vi "Get Child Classes.vi"(8 "error in (no error)":errorcluster, 11 "Test in":refnum<class "Test.lvclass">) -> (0 "error out":errorcluster, 2 "Child Classes":refnum<class "Test.lvclass">[](array[class]))   [LabVIEW 2018, in "Test.lvclass"]
uses:
  Test.lvclass
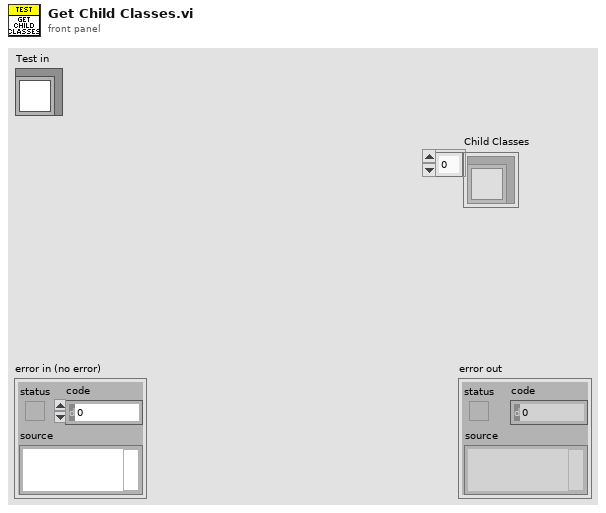
[diagram p1: front panel]
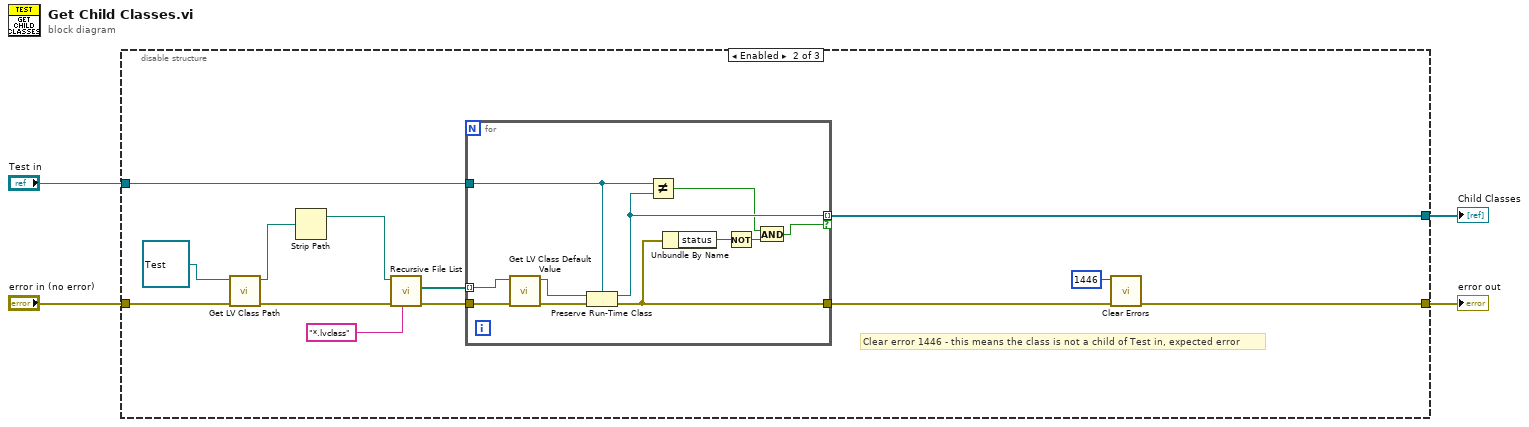
[diagram p0: block diagram]
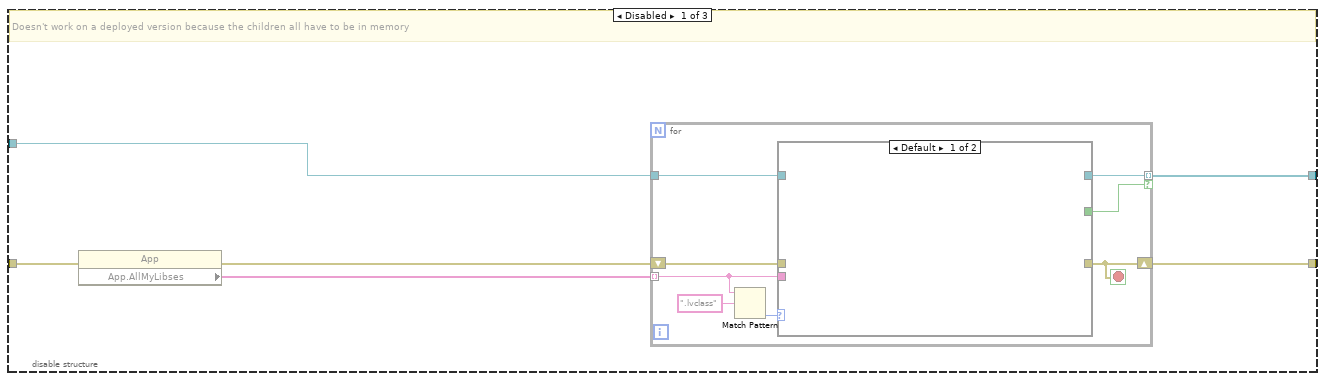
[diagram p2: hidden frame]
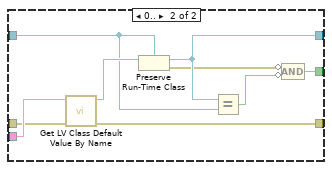
[diagram p3: hidden frame]
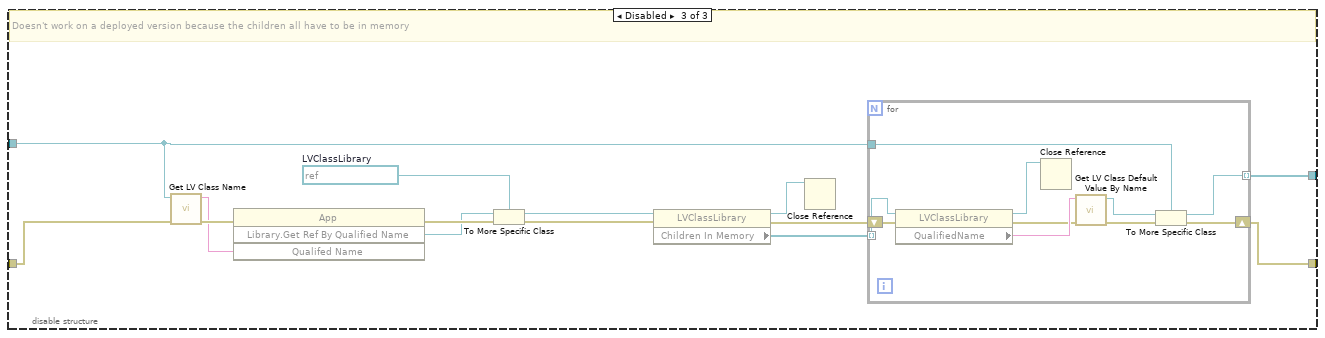
[diagram p4: hidden frame]
diagram:
  n1 = disable-structure shown="Enabled" {
    disable-tunnel: "Test in" -> [w8 w32 w52]
    disable-tunnel: [w7 w31 w53] -> w3
    disable-tunnel: "error in (no error)" -> [w6 w40 w55]
    disable-tunnel: [w5 w29 w54] -> w1
    frame Disabled {
      # "Doesn't work on a deployed version because the children all have to be in memory"
      n2 = property class="App"(error in=w6) -> (error out=w9:errorcluster, "App.AllMyLibses"=w10:string[])  [unwired: 1 in, 1 out]
      n3 = for {
        tunnel: w10 -> [w18] mode=indexing
        tunnel: [w13] -> w7 mode=indexing if=w12
        shift-right: [w14] -> w5
        shift-left: w9 -> [w15]
        tunnel: w8 -> [w11]
        stop <- w14 stop-if-true
        n4 = Match Pattern(string=w18, regular expression=".lvclass") -> (offset past match=w17:i32)  [unwired: 1 in, 3 out]
        n5 = case shown="Default" w17 {
          tunnel: [_ w26] -> w13
          tunnel: w18 -> [_ w23]
          tunnel: [_ w22] -> w12
          tunnel: [_ w21] -> w14
          tunnel: w15 -> [_ w20]
          tunnel: w11 -> [_ w19]
          frame Default {
          }
          frame 0.. {
            n6 = call <vilib>:"Get LV Class Default Value By Name.vi"("error in (no error)"=w20, "class name"=w23) -> ("error out"=w21:errorcluster, "object"=w27:refnum<class>)  [unwired: 8 in]
            n7 = Preserve Run-Time Class(object in=w27, 2:w19) -> (object out=w26:refnum<class "Test.lvclass">, error out=w24:errorcluster)  [unwired: 1 in]
            n8 = Equal?(x=w26, y=w19) -> (x = y?=w25:bool)
            n9 = Compound Arithmetic op=AND(invert w24, invert w25) -> (w22:bool)
          }
        }
      }
    }
    frame Enabled {
      # "Clear error 1446 - this means the class is not a child of Test in, expected error"
      n10 = call <vilib>:"Get LV Class Path.vi"("error in (no error)"=w40, "object"=refnum<class "Test.lvclass"> refnum ("Test.lvclass")) -> ("error out"=w36:errorcluster, "class path"=w39:path)  [unwired: 8 in]
      n11 = Strip Path(path=w39) -> (stripped path=w37:path)  [unwired: 1 out]
      n12 = call <vilib>:"Recursive File List.vi"("pattern"="*.lvclass", "error in (no error)"=w36, "Folder Path"=w37) -> ("error out"=w33:errorcluster, "All Files in Dir"=w34:path[])  [unwired: 4 in, 3 out]
      n13 = for {
        tunnel: w34 -> [w50] mode=indexing
        tunnel: w33 -> [w51]
        tunnel: w32 -> [w44]
        tunnel: [w45] -> w31 mode=indexing if=w41
        tunnel: [w47] -> w30
        n14 = call <vilib>:"Get LV Class Default Value.vi"("error in (no error)"=w51, "class path"=w50) -> ("error out"=w49:errorcluster, "object"=w48:refnum<class>)  [unwired: 8 in]
        n15 = Preserve Run-Time Class(object in=w48, error in=w49, 2:w44) -> (object out=w45:refnum<class "Test.lvclass">, error out=w47:errorcluster)
        n16 = Not Equal?(x=w44, y=w45) -> (x != y?=w42:bool)
        n17 = Unbundle By Name(w47) -> ("status"=w46:bool)
        n18 = Not(x=w46) -> (.not. x?=w43:bool)
        n19 = And(x=w42, y=w43) -> (x .and. y?=w41:bool)
      }
      n20 = call <vilib>:"Clear Errors.vi"("error in (no error)"=w30, "specific error code to clear (0: all)"=1446) -> ("error out"=w29:errorcluster)  [unwired: 4 in, 1 out]
    }
    frame Disabled {
      w56 = refnum<vi> refnum  # LVClassLibrary
      # "Doesn't work on a deployed version because the children all have to be in memory"
      n21 = call <vilib>:"Get LV Class Name.vi"("error in (no error)"=w55, "object"=w52) -> ("error out"=w58:errorcluster, "class name"=w57:string)  [unwired: 8 in]
      n22 = invoke class="App" method="Library.Get Ref By Qualified Name"(error in=w58, "Qualifed Name"=w57) -> (error out=w60:errorcluster, "Library.Get Ref By Qualified Name"=w59:refnum<vi>)  [unwired: 2 in, 2 out]
      n23 = To More Specific Class(target class=w56, reference=w59, error in=w60) -> (specific class reference=w61:refnum<vi>, error out=w62:errorcluster)
      n24 = property class="LVClassLibrary"(reference=w61, error in=w62) -> (reference out=w65:refnum<vi>, error out=w64:errorcluster, "Children In Memory"=w63:refnum<vi>[])
      n25 = Close Reference(reference=w65) -> ()  [unwired: 1 in, 1 out]
      n26 = for {
        tunnel: w63 -> [w75] mode=indexing
        shift-right: [w69] -> w54
        shift-left: w64 -> [w73]
        tunnel: [w67] -> w53 mode=indexing
        tunnel: w52 -> [w66]
        n27 = property class="LVClassLibrary"(reference=w75, error in=w73) -> (reference out=w70:refnum<vi>, error out=w72:errorcluster, "QualifiedName"=w74:string)
        n28 = Close Reference(reference=w70) -> ()  [unwired: 1 in, 1 out]
        n29 = call <vilib>:"Get LV Class Default Value By Name.vi"("error in (no error)"=w72, "class name"=w74) -> ("error out"=w71:errorcluster, "object"=w68:refnum<class>)  [unwired: 8 in]
        n30 = To More Specific Class(target class=w66, reference=w68, error in=w71) -> (specific class reference=w67:refnum<class "Test.lvclass">, error out=w69:errorcluster)
      }
    }
  }
  "error out" <- w1
  "Child Classes" <- w3
